vi "Write Digitizer.vi"(8 "error in (no error)":errorcluster, 10 "Digitizer":refnum<vi>, 11 "Measurement UI in":refnum<class "Measurement UI.lvclass">) -> (0 "error out":errorcluster, 3 "Measurement UI out":refnum<class "Measurement UI.lvclass">)   [LabVIEW 2016, in "Measurement UI.lvlib" / "Measurement UI.lvclass"]
uses:
  Measurement UI.lvclass
  Measurement UI.lvclass/Measurement UI.ctl
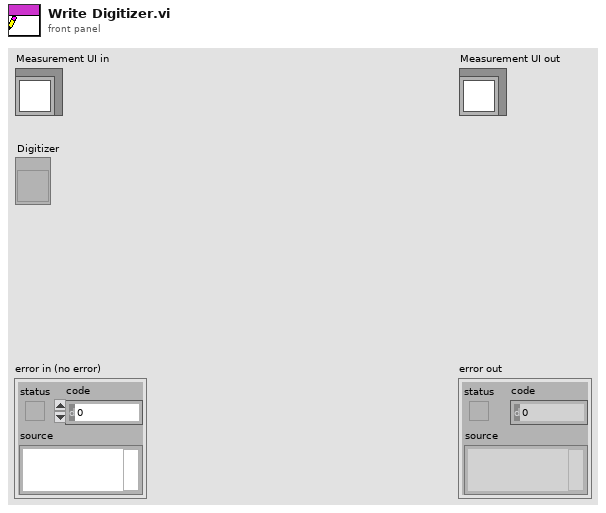
[diagram p1: front panel]
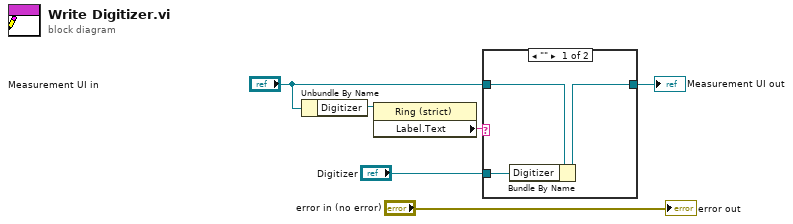
[diagram p0: block diagram]
diagram:
  n1 = Unbundle By Name("Measurement UI in") -> ("Digitizer"=w4:refnum<vi>)
  n2 = property class="Ring (strict)"(reference=w4) -> ("Label.Text"=w2:string)  [unwired: 1 in, 2 out]
  n3 = case shown="\"\"" w2 {
    tunnel: [w8 w10] -> w6
    tunnel: "Measurement UI in" -> [w9 w10]
    tunnel: "Digitizer" -> [w7 _]
    frame "" {
      n4 = Bundle By Name(cluster=w9, "Digitizer"=w7) -> (w8:refnum<class "Measurement UI.lvclass">)
    }
    frame Default {
    }
  }
  "Measurement UI out" <- w6
  "error out" <- "error in (no error)"
